vi "GDC Manuell.vi"() -> ()   [LabVIEW 2020, in "Linearisierung v2.lvlib" / "Gasteiler.lvlib" / "Horiba GDC.lvlib"]
uses:
  Horiba GDC.lvlib
  Visualisierungs Elemente/Button.ctl
  Visualisierungs Elemente/Zahlen-Eingabefeld.ctl
  Visualisierungs Elemente/String - Eingabefeld.ctl
  Visualisierungs Elemente/Zahlen-Ausgabefeld.ctl
  Visualisierungs Elemente/String - Ausgabefeld.ctl
  AK-Schnittstelle/Serielle Parameter.ctl
  Aktionen FGV Gasteiler Daten.ctl
  Aktion Befehl.ctl
  Allgemein/allgemeine Sub-VIs.lvlib
  Gasteiler.lvlib
  AK-Schnittstelle/AK Seriell/AK Seriell.lvlib
panel:
  in  "Schnittstelle":refnum<visa-resource-name>
  in  "Serielle Parameter":T1={"VISA resource name"="COM1", "baud rate"=38400, "data bits"=8, "parity"=0, "stop bits"=10, "flow control"=0} {"flow control" items=["None"=0, "XON/XOFF"=1, "RTS/CTS"=2, "DTR/DSR"=4]; "stop bits" items=["1.0"=10, "1.5"=15, "2.0"=20]; "parity" items=["None", "Odd", "Even", "Mark", "Space"]; "data bits" min=5 max=8 step=1}
  out "Gasteiler Status 2":T2[](array[typedef]) caption="Gasteiler Status"
  out "Störung Kommunikation":bool
  out "Störung Gasteiler":bool
  out "ppm 2":bool
  in  "Start":T3
  in  "Stand By":T3
  out "Gasteiler Status":T2
  out "Konzentration":T4 format="%.3f"
  in  "Teilungsstufe (0-500)":T5 format="%#_5g"
  in  "ppm":bool
  in  "Enum":enum16{"N2", "O2"}(ring)
  out "Gas":string[](array[string])
  in  "Formelzeichen Gas":T6
  in  "Gas Konzentration":T5 format="%#_5g"
  in  "BEENDEN":T3 caption="Exit"
  # "Horiba GDC"
  # "Status"
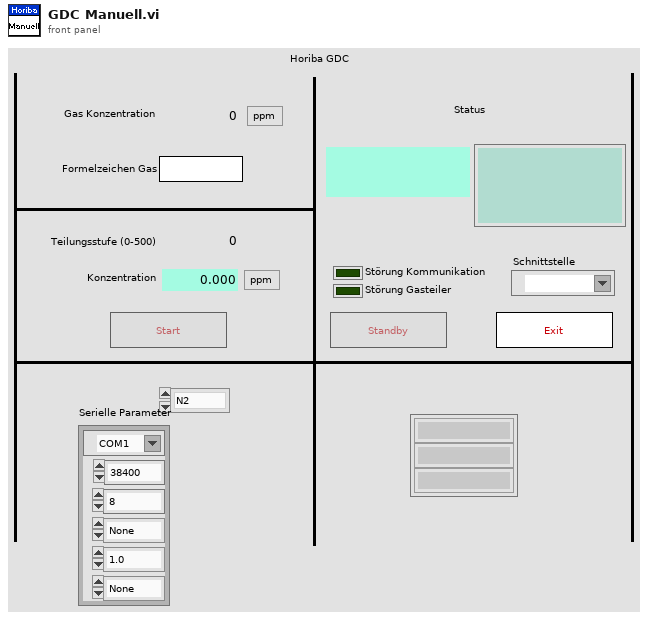
[diagram p1: front panel]
types:
  T1 = typedef "AK-Schnittstelle.lvlib/AK Seriell.lvlib/Serielle Parameter.ctl" = cluster{"VISA resource name":refnum<visa-resource-name>, "baud rate":u32, "data bits":u16, "parity":u16, "stop bits":u16, "flow control":u16}
  T2 = typedef "String - Ausgabefeld.ctl" = string
  T3 = typedef "Button.ctl" = bool
  T4 = typedef "Zahlen-Ausgabefeld.ctl" = sgl
  T5 = typedef "Zahlen-Eingabefeld.ctl" = sgl
  T6 = typedef "String - Eingabefeld.ctl" = string
  T7 = typedef "Linearisierung v2.lvlib/Gasteiler.lvlib/Aktionen FGV Gasteiler Daten.ctl" = enum16{"lesen", "Gasteiler Daten", "Seriellen Param.", "MB-Endwert", "laden", "speichern", "Anforderung", "TCP", "Aufzeichnung Start"}
  T8 = typedef "Linearisierung v2.lvlib/Gasteiler.lvlib/Horiba GDC.lvlib/Aktion Befehl.ctl" = enum16{"lesen", "initialisieren", "Beenden", "Standby", "GD/CC", "Info", "Flow", "Alarm", "GD parameter", "GD point", "Durchfluss", "Spuelen1", "Spuelen1 On", "Spuelen1Off", "Spuelen2", "Ventil-Abfrage", "Reset"}
  T9 = enum8{"Enabled", "Disabled", "Disabled and Grayed Out"}
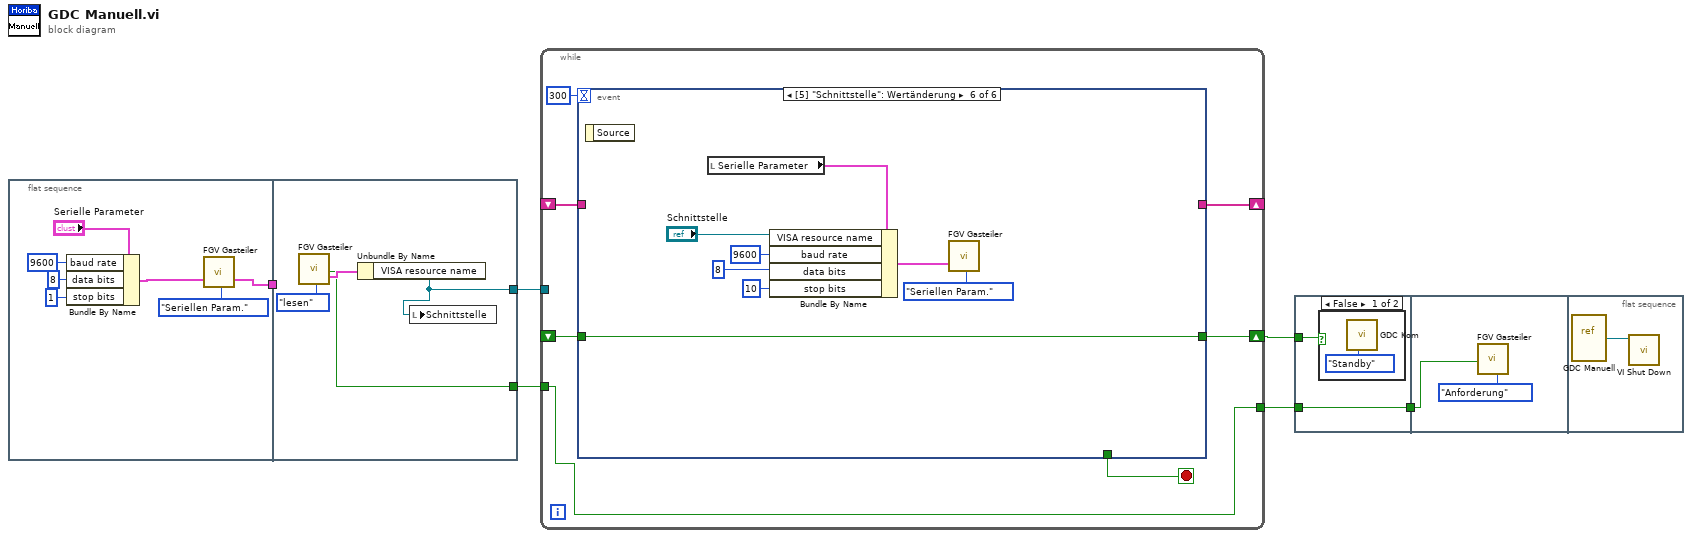
[diagram p0: block diagram]
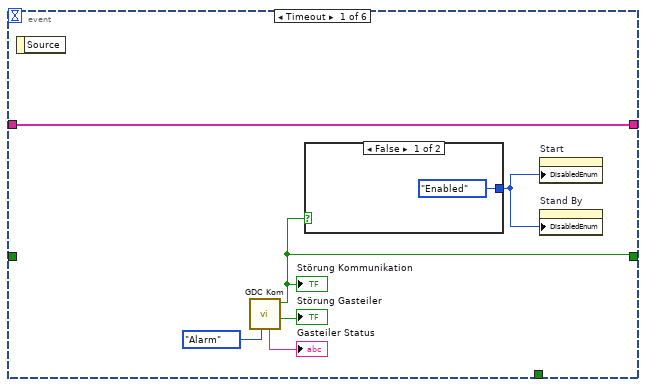
[diagram p3: hidden frame]
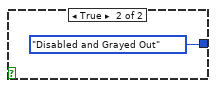
[diagram p4: hidden frame]
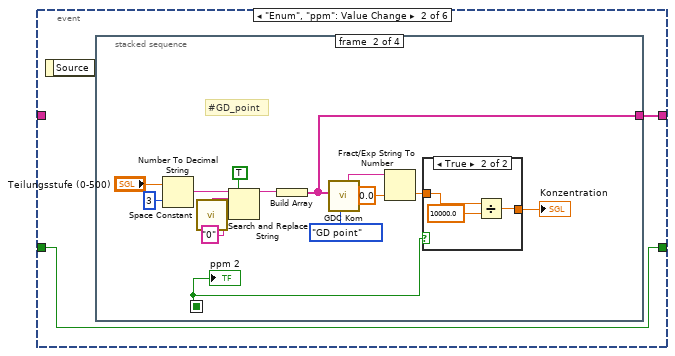
[diagram p5: hidden frame]
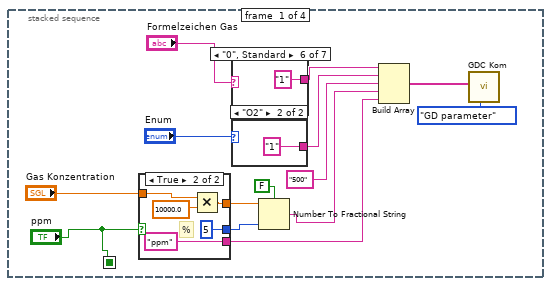
[diagram p6: hidden frame]
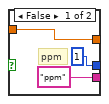
[diagram p7: hidden frame]
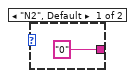
[diagram p8: hidden frame]
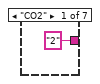
[diagram p9: hidden frame]
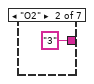
[diagram p10: hidden frame]
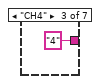
[diagram p11: hidden frame]
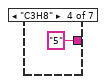
[diagram p12: hidden frame]
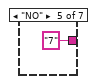
[diagram p13: hidden frame]
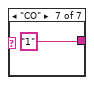
[diagram p14: hidden frame]
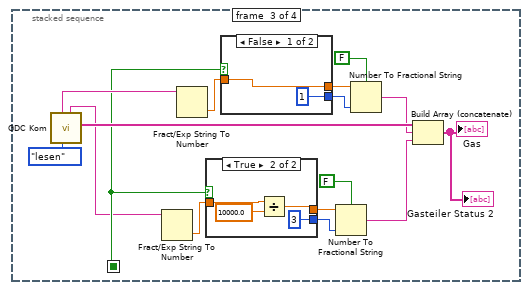
[diagram p16: hidden frame]
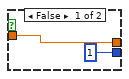
[diagram p17: hidden frame]
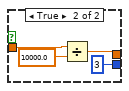
[diagram p18: hidden frame]
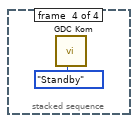
[diagram p19: hidden frame]
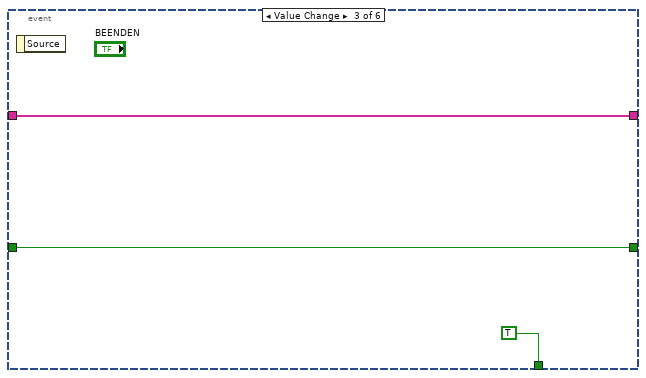
[diagram p20: hidden frame]
diagram:
  n1 = flat-sequence {
    tunnel: [w7] -> w5
    tunnel: w5 -> [_]
    tunnel: [w15] -> w4
    tunnel: [w14] -> w3
    frame #0 {
      n2 = Bundle By Name(cluster="Serielle Parameter", "baud rate"=u32 9600, "data bits"=u16 8, "stop bits"=u16 1) -> (w11:T1)
      n3 = call "FGV Gasteiler.vi"("Serielle Parameter"=w11, "Aktionen"=Aktionen_FGV_Gasteiler_Daten."Seriellen Param.") -> ("Serielle Parameter"=w7:T1)  [unwired: 10 in, 7 out]
    }
    frame #1 {
      n4 = call "FGV Gasteiler.vi"("Aktionen"=Aktionen_FGV_Gasteiler_Daten."lesen") -> ("Anforderung"=w14:bool, "Serielle Parameter"=w16:T1)  [unwired: 11 in, 6 out]
      n5 = Unbundle By Name(w16) -> ("VISA resource name"=w15:refnum<visa-resource-name>)
      n6 = local write "Schnittstelle"(w15) -> ()
    }
  }
  n7 = while {
    shift-right: [w22] -> _
    shift-left: _ -> [w21]
    shift-right: [w20] -> w6
    shift-left: _ -> [w19]
    tunnel: w4 -> [_]
    tunnel: w3 -> [w18]
    tunnel: [w18] -> w2
    stop <- w23 stop-if-true
    n8 = event shown="[5] \"Schnittstelle\": Wertänderung" {
      selector: _ -> [_ _ _ _ _ _]
      dyn-events: _ -> [_ _ _ _ _ _]
      timeout: 300 -> [_ _ _ _ _ _]
      tunnel: [_ _ TRUE _ _ _] -> w23
      tunnel: [w28 w34 w114 _ _ _] -> w22
      tunnel: w21 -> [w28 _ w114 w117 _ _]
      tunnel: [w25 w33 w113 w116 w119 w124] -> w20
      tunnel: w19 -> [_ w33 w113 w116 w119 w124]
      event Timeout {
        n9 = event-data() -> ()  [unwired: 1 in, 1 out]
        n10 = call "GDC Kom.vi"("Befehl"=Aktion_Befehl."Alarm") -> ("Status (alarm)"=→"Störung Gasteiler":bool, "Fehler"=w25:bool, "Status"=→"Gasteiler Status":string)  [unwired: 4 in, 4 out]
        "Störung Kommunikation" <- w25
        n11 = case shown="False" w25 {
          tunnel: [T9."Enabled" ("Deaktiviert") T9."Disabled and Grayed Out" ("Deaktiviert")] -> w26
          frame False {
          }
          frame True {
          }
        }
        n12 = property on="Start" class="Bool."("DisabledEnum"=w26) -> ()  [unwired: 2 in, 2 out]
        n13 = property on="Stand By" class="Bool."("DisabledEnum"=w26) -> ()  [unwired: 2 in, 2 out]
      }
      event "Enum", "ppm": Value Change {
        n14 = event-data() -> ()  [unwired: 1 in, 1 out]
        n15 = stacked-sequence {
          seq-local: ["ppm" _ _ _] -> [_ w72 w86 _]
          tunnel: [_ w73 _ _] -> w34
          frame #0 {
            n16 = case shown="True" "ppm" {
              tunnel: [i16 1 ("Genauigkeit (6)") i16 5 ("Genauigkeit (6)")] -> w38
              tunnel: "Gas Konzentration" -> [w50 w55]
              tunnel: [w50 w54] -> w39
              tunnel: ["ppm" "ppm"] -> w35
              frame False {
                # "ppm"
              }
              frame True {
                # "%"
                n17 = Multiply(x=w55, y=T5 10000.0) -> (x*y=w54:T5)
              }
            }
            n18 = case shown="\"0\", Standard" "Formelzeichen Gas" {
              tunnel: ["2" "3" "4" "5" "7" "1" "1"] -> w46
              frame "CO2" {
              }
              frame "O2" {
              }
              frame "CH4" {
              }
              frame "C3H8" {
              }
              frame "NO" {
              }
              frame "0", Default {
              }
              frame "CO" {
              }
            }
            n19 = case shown="\"O2\"" "Enum" {
              tunnel: ["0" "1"] -> w45
              frame "N2", Default {
              }
              frame "O2" {
              }
            }
            n20 = Number To Fractional String(use system decimal point (T)=FALSE ("Systemdezimalzeichen verwenden (T)"), number=w39, precision (6)=w38) -> (F-format string=w37:string)  [unwired: 1 in]
            n21 = Build Array(w46, w45, "500", w37, w35) -> (w43:string[])
            n22 = call "GDC Kom.vi"("Befehl"=Aktion_Befehl."GD parameter", "Daten"=w43) -> ()  [unwired: 3 in, 7 out]
          }
          frame #1 {
            # "#GD_point"
            n23 = Number To Decimal String(number="Teilungsstufe (0-500)", width (-)=i16 3 ("Breite (-)")) -> (decimal integer string=w67:string)
            n24 = call <vilib>:"Space Constant.vi"() -> ("String"=w69:string)
            n25 = Search and Replace String(replace all?=TRUE ("Alle ersetzen? (F)"), input string=w67, search string=w69, replace string="0" ("Ersetzungs-String (\"\")")) -> (result string=w66:string)  [unwired: 4 in, 3 out]
            n26 = Build Array(w66) -> (w73:string[])
            n27 = call "GDC Kom.vi"("Befehl"=Aktion_Befehl."GD point", "Daten"=w73) -> ("Konzentration"=w78:string)  [unwired: 3 in, 6 out]
            n28 = Fract/Exp String To Number(string=w78, default (0 dbl)=sgl 0.0 ("Standard (0 I32)")) -> (number=w75:sgl)  [unwired: 2 in, 1 out]
            n29 = case shown="True" w72 {
              tunnel: w75 -> [w80 w82]
              tunnel: [w80 w83] -> w74
              frame False {
              }
              frame True {
                n30 = Divide(x=w82, y=sgl 10000.0) -> (x/y=w83:sgl)
              }
            }
            "Konzentration" <- w74
            "ppm 2" <- w72
          }
          frame #2 {
            n31 = call "GDC Kom.vi"("Befehl"=Aktion_Befehl."lesen") -> ("Gas"=w98:string[], "Konzentration"=w85:string, "Konzentration 2"=w97:string)  [unwired: 4 in, 4 out]
            n32 = Fract/Exp String To Number(string=w85) -> (number=w87:dbl)  [unwired: 3 in, 1 out]
            n33 = Fract/Exp String To Number(string=w97) -> (number=w96:dbl)  [unwired: 3 in, 1 out]
            n34 = case shown="True" w86 {
              tunnel: w87 -> [w101 w104]
              tunnel: [w101 w105] -> w88
              tunnel: [i16 1 ("Genauigkeit (6)") i16 3 ("Genauigkeit (6)")] -> w89
              frame False {
              }
              frame True {
                n35 = Divide(x=w104, y=10000.0) -> (x/y=w105:dbl)
              }
            }
            n36 = case shown="False" w86 {
              tunnel: w96 -> [w107 w110]
              tunnel: [w107 w111] -> w95
              tunnel: [i16 1 ("Genauigkeit (6)") i16 3 ("Genauigkeit (6)")] -> w93
              frame False {
              }
              frame True {
                n37 = Divide(x=w110, y=10000.0) -> (x/y=w111:dbl)
              }
            }
            n38 = Number To Fractional String(use system decimal point (T)=FALSE ("Systemdezimalzeichen verwenden (T)"), number=w88, precision (6)=w89) -> (F-format string=w84:string)  [unwired: 1 in]
            n39 = Number To Fractional String(use system decimal point (T)=FALSE ("Systemdezimalzeichen verwenden (T)"), number=w95, precision (6)=w93) -> (F-format string=w94:string)  [unwired: 1 in]
            n40 = Build Array (concatenate)(w98, w94, w84) -> (→"Gas" →"Gasteiler Status 2":string[])
          }
          frame #3 {
            n41 = call "GDC Kom.vi"("Befehl"=Aktion_Befehl."Standby") -> ()  [unwired: 4 in, 7 out]
          }
        }
      }
      event Value Change {
        n42 = event-data() -> ()  [unwired: 1 in, 1 out]
      }
      event Value Change {
        n43 = event-data() -> ()  [unwired: 1 in, 1 out]
        n44 = call "GDC Kom.vi"("Befehl"=Aktion_Befehl."GD point", "Daten"=w117) -> ()  [unwired: 3 in, 7 out]
      }
      event Value Change {
        n45 = event-data() -> ()  [unwired: 1 in, 1 out]
        n46 = call "GDC Kom.vi"("Befehl"=Aktion_Befehl."Standby") -> ()  [unwired: 4 in, 7 out]
      }
      event "Schnittstelle": Value Change {
        n47 = event-data() -> ()  [unwired: 1 in, 1 out]
        n48 = local read "Serielle Parameter"() -> (w125:T1)
        n49 = Bundle By Name(cluster=w125, "VISA resource name"="Schnittstelle", "baud rate"=u32 9600, "data bits"=u16 8, "stop bits"=u16 10) -> (w128:T1)
        n50 = call "FGV Gasteiler.vi"("Serielle Parameter"=w128, "Aktionen"=Aktionen_FGV_Gasteiler_Daten."Seriellen Param.") -> ()  [unwired: 10 in, 8 out]
      }
    }
  }
  n51 = flat-sequence {
    tunnel: w6 -> [w130]
    tunnel: w2 -> [w129]
    tunnel: [w129] -> w1
    tunnel: w1 -> [w132]
    frame #0 {
      n52 = case shown="False" w130 {
        frame False {
          n53 = call "GDC Kom.vi"("Befehl"=Aktion_Befehl."Standby") -> ()  [unwired: 4 in, 7 out]
        }
        frame True {
        }
      }
    }
    frame #1 {
      n54 = call "FGV Gasteiler.vi"("Anforderung"=w132, "Aktionen"=Aktionen_FGV_Gasteiler_Daten."Anforderung") -> ()  [unwired: 10 in, 8 out]
    }
    frame #2 {
      n55 = vi-ref "GDC Manuell.vi"() -> (w134:refnum<vi>)
      n56 = call "VI Shut Down.vi"("VI Referenz"=w134) -> ()  [unwired: 11 in]
    }
  }
